vi "DrawCrossHairs.vi"(11 "Image In":T1) -> (3 "Image Out":T1)   [LabVIEW 2012]
uses:
  <vilib>/vision/Image Controls.llb/IMAQ Image.ctl
  <vilib>/vision/NI_Vision_Development_Module.lvlib
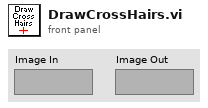
[diagram p1: front panel]
types:
  T1 = typedef "IMAQ Image.ctl" = refnum<image>
  T2 = cluster{"Red or Hue value":u8, "Green or Sat value":u8, "Blue or Luma or Val or Inten value":u8}
  T3 = cluster{dbl, "Blue or Luma or Val or Inten value":u8}
  T4 = cluster{"Blue or Luma or Val or Inten value":u8, dbl}
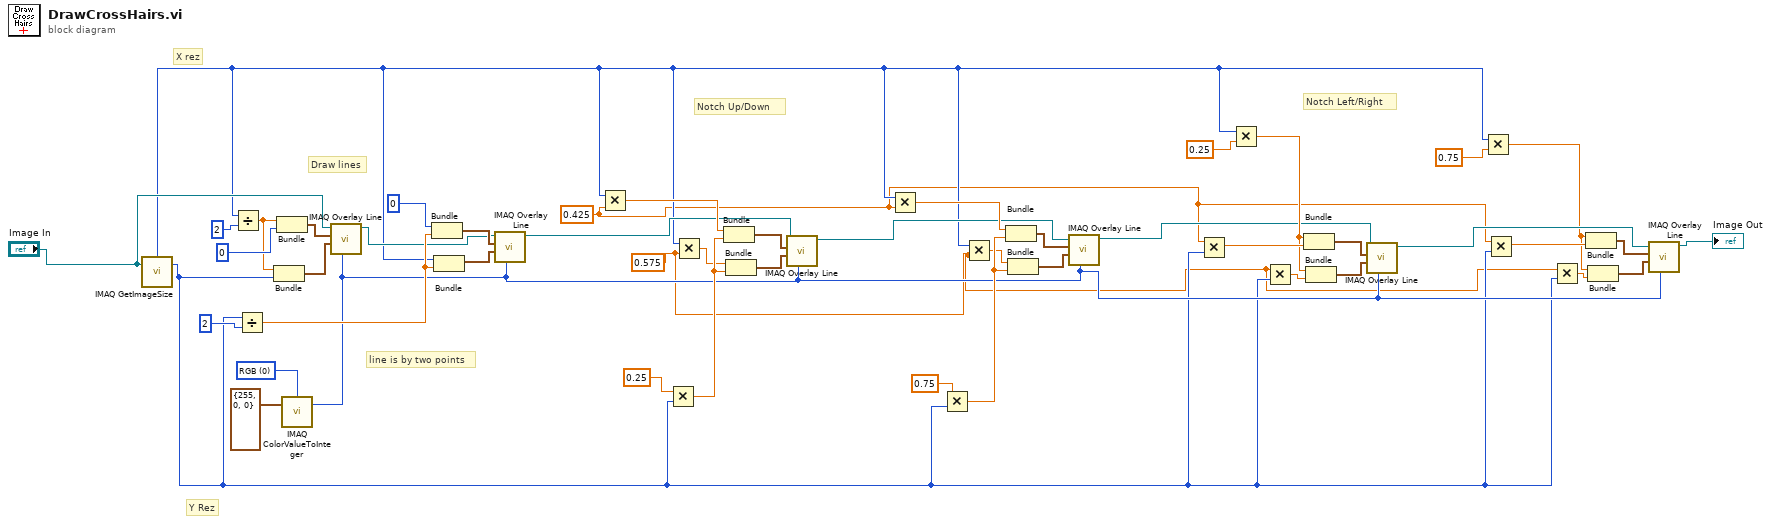
[diagram p0: block diagram]
diagram:
  w1 = 0.575
  w2 = 0.425
  w46 = u16 0 items=["RGB", "HSL", "HSV", "HSI"] ("Color Mode")
  # "Notch Left/Right"
  # "Y Rez"
  # "X rez"
  # "Notch Up/Down"
  # "Draw lines"
  # "line is by two points"
  n1 = call "IMAQ GetImageSize"("Image"="Image In") -> ("Y Resolution"=w9:i32, "X Resolution"=w10:i32)  [unwired: 3 in, 1 out]
  n2 = Divide(x=w10, y=2) -> (x/y=w41:dbl)
  n3 = Divide(x=w9, y=2) -> (x/y=w36:dbl)
  n4 = Bundle(w41, "Y Resolution"=w9) -> (w40:cluster{dbl, "Y Resolution":i32})  [unwired: 1 in]
  n5 = Bundle(w41, "Blue or Luma or Val or Inten value"=u8 0) -> (w43:T3)  [unwired: 1 in]
  n6 = call "IMAQ ColorValueToInteger"("Color Value"=T2 {"Red or Hue value"=255, "Green or Sat value"=0, "Blue or Luma or Val or Inten value"=0}, "Color Mode"=w46) -> ("U32 value"=w19:u32)  [unwired: 3 in, 3 out]
  n7 = call "IMAQ Overlay Line"("Color"=w19, "End Point"=w40, "Start Point"=w43, "Image"="Image In") -> ("Image Out"=w35:T1)  [unwired: 6 in, 1 out]
  n8 = Bundle("Blue or Luma or Val or Inten value"=u8 0, w36) -> (w39:T4)  [unwired: 1 in]
  n9 = Bundle("X Resolution"=w10, w36) -> (w38:cluster{"X Resolution":i32, dbl})  [unwired: 1 in]
  n10 = call "IMAQ Overlay Line"("Color"=w19, "End Point"=w38, "Start Point"=w39, "Image"=w35) -> ("Image Out"=w26:T1)  [unwired: 6 in, 1 out]
  n11 = Multiply(x=w10, y=w2) -> (x*y=w29:dbl)
  n12 = Multiply(x=0.25, y=w9) -> (x*y=w31:dbl)
  n13 = Multiply(x=w10, y=w1) -> (x*y=w30:dbl)
  n14 = Bundle(w29, w31) -> (w28:cluster{dbl, dbl})  [unwired: 1 in]
  n15 = Bundle(w30, w31) -> (w27:cluster{dbl, dbl})  [unwired: 1 in]
  n16 = call "IMAQ Overlay Line"("Color"=w19, "End Point"=w27, "Start Point"=w28, "Image"=w26) -> ("Image Out"=w23:T1)  [unwired: 6 in, 1 out]
  n17 = Multiply(x=w10, y=w2) -> (x*y=w24:dbl)
  n18 = Multiply(x=0.75, y=w9) -> (x*y=w32:dbl)
  n19 = Multiply(x=w10, y=w1) -> (x*y=w25:dbl)
  n20 = Bundle(w24, w32) -> (w22:cluster{dbl, dbl})  [unwired: 1 in]
  n21 = Bundle(w25, w32) -> (w21:cluster{dbl, dbl})  [unwired: 1 in]
  n22 = call "IMAQ Overlay Line"("Color"=w19, "End Point"=w21, "Start Point"=w22, "Image"=w23) -> ("Image Out"=w4:T1)  [unwired: 6 in, 1 out]
  n23 = Multiply(x=w2, y=w9) -> (x*y=w12:dbl)
  n24 = Multiply(x=w10, y=0.25) -> (x*y=w11:dbl)
  n25 = Multiply(x=w1, y=w9) -> (x*y=w13:dbl)
  n26 = Bundle(w11, w12) -> (w8:cluster{dbl, dbl})  [unwired: 1 in]
  n27 = Bundle(w11, w13) -> (w7:cluster{dbl, dbl})  [unwired: 1 in]
  n28 = call "IMAQ Overlay Line"("Color"=w19, "End Point"=w7, "Start Point"=w8, "Image"=w4) -> ("Image Out"=w20:T1)  [unwired: 6 in, 1 out]
  n29 = Multiply(x=w10, y=0.75) -> (x*y=w14:dbl)
  n30 = Multiply(x=w2, y=w9) -> (x*y=w17:dbl)
  n31 = Multiply(x=w1, y=w9) -> (x*y=w18:dbl)
  n32 = Bundle(w14, w17) -> (w6:cluster{dbl, dbl})  [unwired: 1 in]
  n33 = Bundle(w14, w18) -> (w5:cluster{dbl, dbl})  [unwired: 1 in]
  n34 = call "IMAQ Overlay Line"("Color"=w19, "End Point"=w5, "Start Point"=w6, "Image"=w20) -> ("Image Out"=→"Image Out":T1)  [unwired: 6 in, 1 out]
